vi "Popup Menu Close.vi"(11 "Error In":errorcluster) -> (15 "Error Out":errorcluster)   [LabVIEW 2020]
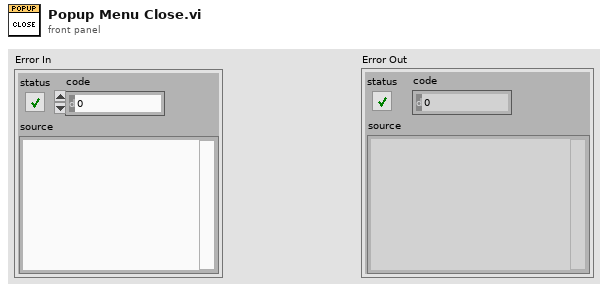
[diagram p1: front panel]
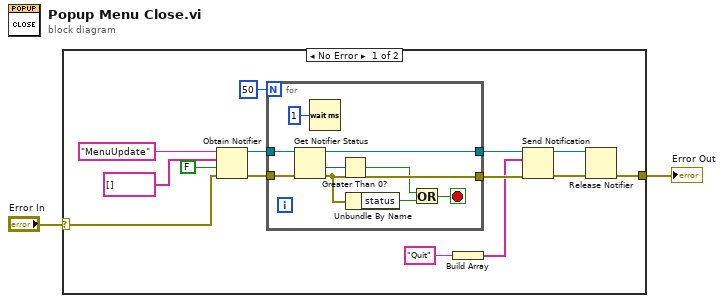
[diagram p0: block diagram]
diagram:
  n1 = case shown="No Error" "Error In" {
    selector: "Error In" -> [w5 w26]
    tunnel: [w6 w26] -> w2
    frame No Error {
      n2 = Obtain Notifier(name (unnamed)="MenuUpdate", notification data type=string[] [], create if not found? (T)=FALSE, error in (no error)=w5) -> (notifier out=w13:refnum<notifier>, error out=w12:errorcluster)  [unwired: 1 out]
      n3 = for {
        N: 50 -> [_]
        tunnel: w13 -> [w25]
        tunnel: w12 -> [w24]
        tunnel: [w22] -> w10
        tunnel: [w20] -> w9
        stop <- w19 stop-if-true
        n4 = Get Notifier Status(notifier=w25, error in (no error)=w24) -> (notifier out=w22:refnum<notifier>, # waiting=w23:i32, error out=w20:errorcluster)  [unwired: 2 out]
        n5 = Wait (ms)(milliseconds to wait=u32 1) -> ()  [unwired: 1 out]
        n6 = Greater Than 0?(x=w23) -> (x > 0?=w18:bool)
        n7 = Unbundle By Name(w20) -> ("status"=w17:bool)
        n8 = Or(x=w18, y=w17) -> (x .or. y?=w19:bool)
      }
      n9 = Build Array("Quit") -> (w3:string[])
      n10 = Send Notification(notification=w3, notifier=w10, error in (no error)=w9) -> (notifier out=w8:refnum<notifier>, error out=w7:errorcluster)
      n11 = Release Notifier(notifier=w8, error in (no error)=w7) -> (error out=w6:errorcluster)  [unwired: 1 in, 2 out]
    }
    frame Error {
    }
  }
  "Error Out" <- w2
